vi "oddeven.vi"() -> ()   [LabVIEW 2024]
uses:
  <vilib>/numeric/Random Number (Range) U64.vi
  <vilib>/numeric/sub_Random U32.vi
panel:
  out "String":string
  out "number":u64
  out "number mod 2":u64
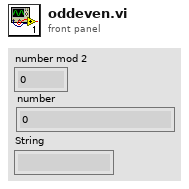
[diagram p1: front panel]
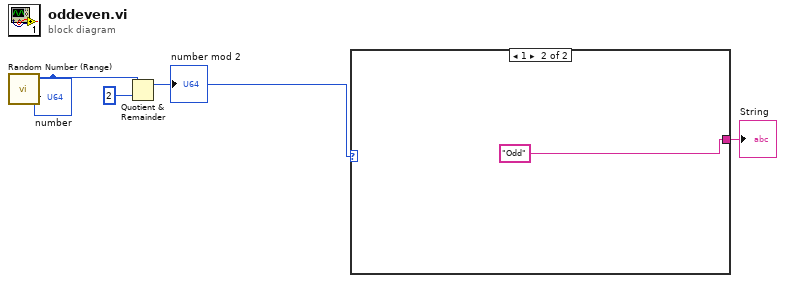
[diagram p0: block diagram]
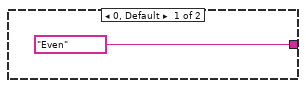
[diagram p2: hidden frame]
diagram:
  n1 = call-poly <vilib>:"Random Number (Range).vi"() -> ("number"=w4:u64)  [unwired: 11 in]
  "number" <- w4
  n2 = Quotient & Remainder(x=w4, y=u64 2) -> (x-y*floor(x/y)=w2:u64)  [unwired: 1 out]
  "number mod 2" <- w2
  n3 = case shown="1" w2 {
    tunnel: ["Even" "Odd"] -> w1
    frame 0, Default {
    }
    frame 1 {
    }
  }
  "String" <- w1
